vi "Craigslist Textbooks for Fusion Table V2.vi"() -> ()   [LabVIEW 2010]
uses:
  <vilib>/Utility/file.llb/Read From Spreadsheet File (string).vi
  <vilib>/Utility/file.llb/Write To Spreadsheet File (string).vi
panel:
  out "File Save Path":string
  out "Array":string[][](array[string])
  out "user books per city":string[][](array[string])
  out "Final filtered":string[][](array[string])
  out "element":string
  out "All closest city data":string[](array[string])
  out "All Data":string[][](array[string])
  out "ID number":string
  in  "Geo Locations 2":string[][](array[string])=[["http://boulder.craigslist.org/bks/", "http://boulder.craigslist.org/bks/index100.html", "http://boulder.craigslist.org/bks/index200.html", "http://boulder.craigslist.org/bks/index300.html", "http://boulder.craigslist.org/bks/index400.html", "http://boulder.craigslist.org/bks/index500.html", "http://boulder.craigslist.org/bks/index600.html", "http://boulder.craigslist.org/bks/index700.html", "http://boulder.craigslist.org/bks/index800.html", "http://boulder.craigslist.org/bks/index900.html", "40.006846", "-105.271575", "CU Boulder", "Boulder", "CO", "4/30/2004 7:48:47 PM", "3558694"], ["http://phoenix.craigslist.org/bks/", "http://phoenix.craigslist.org/bks/index100.html", "http://phoenix.craigslist.org/bks/index200.html", "http://phoenix.craigslist.org/bks/index300.html", "http://phoenix.craigslist.org/bks/index400.html", "http://phoenix.craigslist.org/bks/index500.html", "http://phoenix.craigslist.org/bks/index600.html", "http://phoenix.craigslist.org/bks/index700.html", "http://phoenix.craigslist.org/bks/index800.html", "http://phoenix.craigslist.org/bks/index900.html", "33.416147", "-111.938152", "ASU Arizona State University", "Phoenix", "AZ", "4/30/2004 7:48:47 PM", "3558688"], ["http://orlando.craigslist.org/bks/", "http://orlando.craigslist.org/bks/index100.html", "http://orlando.craigslist.org/bks/index200.html", "http://orlando.craigslist.org/bks/index300.html", "http://orlando.craigslist.org/bks/index400.html", "http://orlando.craigslist.org/bks/index500.html", "http://orlando.craigslist.org/bks/index600.html", "http://orlando.craigslist.org/bks/index700.html", "http://orlando.craigslist.org/bks/index800.html", "http://orlando.craigslist.org/bks/index900.html", "28.602326", "-81.19994", "UCF University of Central Florida", "orlando", "FL", "", "3558796"], ["http://austin.craigslist.org/bks/", "http://austin.craigslist.org/bks/index100.html", "http://austin.craigslist.org/bks/index200.html", "http://austin.craigslist.org/bks/index300.html", "http://austin.craigslist.org/bks/index400.html", "http://austin.craigslist.org/bks/index500.html", "http://austin.craigslist.org/bks/index600.html", "http://austin.craigslist.org/bks/index700.html", "http://austin.craigslist.org/bks/index800.html", "http://austin.craigslist.org/bks/index900.html", "30.28629", "-97.740211", "UT Austin University of Texas at Austin", "Austin", "TX", "40.006846", "3588692"], ["http://columbus.craigslist.org/bks/", "http://columbus.craigslist.org/bks/index100.html", "http://columbus.craigslist.org/bks/index200.html", "http:/columbus.craigslist.org/bks/index300.html", "http://columbus.craigslist.org/bks/index400.html", "http://columbus.craigslist.org/bks/index500.html", "http://columbus.craigslist.org/bks/index600.html", "http://columbus.craigslist.org/bks/index700.html", "http://columbus.craigslist.org/bks/index800.html", "http://columbus.craigslist.org/bks/index900.html", "40.000778", "-83.010421", "OSU Ohio State University", "Columbus", "OH", "4/30/2004 7:48:47 PM", "3558876"], ["http://minneapolis.craigslist.org/bks/", "http://minneapolis.craigslist.org/bks/index100.html", "http://minneapolis.craigslist.org/bks/index200.html", "http://minneapolis.craigslist.org/bks/index300.html", "http://minneapolis.craigslist.org/bks/index400.html", "http://minneapolis.craigslist.org/bks/index500.html", "http://minneapolis.craigslist.org/bks/index600.html", "http://minneapolis.craigslist.org/bks/index700.html", "http://minneapolis.craigslist.org/bks/index800.html", "http://minneapolis.craigslist.org/bks/index900.html", "44.974999", "-93.231847", "U of M University of Minnesota", "minneapolis", "MN", "", "3558694"], ["http://losangeles.craigslist.org/lac/bks/", "http://losangeles.craigslist.org/lac/bks/index100.html", "http://losangeles.craigslist.org/lac/bks/index200.html", "http://losangeles.craigslist.org/lac/bks/index300.html", "http://losangeles.craigslist.org/lac/bks/index400.html", "http://losangeles.craigslist.org/lac/bks/index500.html", "http://losangeles.craigslist.org/lac/bks/index600.html", "http://losangeles.craigslist.org/lac/bks/index700.html", "http://losangeles.craigslist.org/lac/bks/index800.html", "http://losangeles.craigslist.org/lac/bks/index900.html", "34.020612", "-118.284409", "USC University of Southern California", "USC", "CA", "40.006846", "3588399"], ["http://boston.craigslist.org/gbs/bks/", "http://boston.craigslist.org/gbs/bks/index100.html", "http://boston.craigslist.org/gbs/bks/index200.html", "http://boston.craigslist.org/gbs/bks/index300.html", "http://boston.craigslist.org/gbs/bks/index400.html", "http://boston.craigslist.org/gbs/bks/index500.html", "http://boston.craigslist.org/gbs/bks/index600.html", "http://boston.craigslist.org/gbs/bks/index700.html", "http://boston.craigslist.org/gbs/bks/index800.html", "http://boston.craigslist.org/gbs/bks/index900.html", "42.372852", "-71.117581", "Harvard University", "Cambridge", "MA", "40.006846", "3589108"], ["http://newhaven.craigslist.org/bks/", "http://newhaven.craigslist.org/bks/index100.html", "http://newhaven.craigslist.org/bks/index200.html", "http://newhaven.craigslist.org/bks/index300.html", "http://newhaven.craigslist.org/bks/index400.html", "http://newhaven.craigslist.org/bks/index500.html", "http://newhaven.craigslist.org/bks/index600.html", "http://newhaven.craigslist.org/bks/index700.html", "http://newhaven.craigslist.org/bks/index800.html", "http://newhaven.craigslist.org/bks/index900.html", "41.311211", "-72.928662", "Yale University", "New Haven", "CT", "40.006846", "3588844"], ["http://sfbay.craigslist.org/pen/bks/", "http://sfbay.craigslist.org/pen/bks/index100.html", "http://sfbay.craigslist.org/pen/bks/index200.html", "http://sfbay.craigslist.org/pen/bks/index300.html", "http://sfbay.craigslist.org/pen/bks/index400.html", "http://sfbay.craigslist.org/pen/bks/index500.html", "http://sfbay.craigslist.org/pen/bks/index600.html", "http://sfbay.craigslist.org/pen/bks/index700.html", "http://sfbay.craigslist.org/pen/index800.html", "http://sfbay.craigslist.org/pen/bks/index900.html", "37.425576", "-122.168891", "Stanford University", "Redwood City", "CA", "40.006846", "3588839"], ["http://chicago.craigslist.org/nch/bks/", "http://chicago.craigslist.org/nch/bks/index100.html", "http://chicago.craigslist.org/nch/bks/index200.html", "http://chicago.craigslist.org/nch/bks/index300.html", "http://chicago.craigslist.org/nch/bks/index400.html", "http://chicago.craigslist.org/nch/bks/index500.html", "http://chicago.craigslist.org/nch/bks/index600.html", "http://chicago.craigslist.org/nch/bks/index700.html", "http://chicago.craigslist.org/nch/bks/index800.html", "http://chicago.craigslist.org/nch/bks/index900.html", "42.057801", "-87.67563", "NU Northwestern University", "Evanston", "IL", "40.006846", "3588099"], ["http://sfbay.craigslist.org/eby/bks/", "http://sfbay.craigslist.org/eby/bks/index100.html", "http://sfbay.craigslist.org/eby/bks/index200.html", "http://sfbay.craigslist.org/eby/bks/index300.html", "http://sfbay.craigslist.org/eby/bks/index400.html", "http://sfbay.craigslist.org/eby/bks/index500.html", "http://sfbay.craigslist.org/eby/bks/index600.html", "http://sfbay.craigslist.org/eby/bks/index700.html", "http://sfbay.craigslist.org/eby/bks/index800.html", "http://sfbay.craigslist.org/eby/bks/index900.html", "37.872296", "-122.258799", "UC Berkeley University of California at Berkeley", "Berkeley", "CA", "40.006846", "3588671"], ["http://fortcollins.craigslist.org/bks/", "http://fortcollins.craigslist.org/bks/index100.html", "http://fortcollins.craigslist.org/bks/index200.html", "http://fortcollins.craigslist.org/bks/index300.html", "http://fortcollins.craigslist.org/bks/index400.html", "http://fortcollins.craigslist.org/bks/index500.html", "http://fortcollins.craigslist.org/bks/index600.html", "http://fortcollins.craigslist.org/bks/index700.html", "http://fortcollins.craigslist.org/bks/index800.html", "http://fortcollins.craigslist.org/bks/index900.html", "40.571556", "-105.080624", "CSU Colorado State University", "Fort Collins", "CO", "40.006846", "3589102"], ["http://denver.craigslist.org/bks/", "http://denver.craigslist.org/bks/index100.html", "http://denver.craigslist.org/bks/index200.html", "http://denver.craigslist.org/bks/index300.html", "http://denver.craigslist.org/bks/index400.html", "http://denver.craigslist.org/bks/index500.html", "http://denver.craigslist.org/bks/index600.html", "http://denver.craigslist.org/bks/index700.html", "http://denver.craigslist.org/bks/index800.html", "http://denver.craigslist.org/bks/index900.html", "39.676707", "-104.962628", "DU University of Denver", "Denver", "CO", "40.006846", "3588279"], ["http://boston.craigslist.org/gbs/bks/", "http://boston.craigslist.org/gbs/bks/index100.html", "http://boston.craigslist.org/gbs/bks/index200.html", "http://boston.craigslist.org/gbs/bks/index300.html", "http://boston.craigslist.org/gbs/bks/index400.html", "http://boston.craigslist.org/gbs/bks/index500.html", "http://boston.craigslist.org/gbs/bks/index600.html", "http://boston.craigslist.org/gbs/bks/index700.html", "http://boston.craigslist.org/gbs/bks/index800.html", "http://boston.craigslist.org/gbs/bks/index900.html", "42.361556", "-71.090759", "MIT Massachusetts Institute of Technology", "Cambridge", "MA", "40.006846", "3588278"]]
  out "Finished Array":string[][](array[string])
  out "One Row Edited":string[](array[string])
  out "Craigslist Link":string
  out "Place":string
  out "One Row Unedited":string[](array[string])
  out "Category":string
  out "Extra Information":string
  out "Price":string
  out "General Location":string
  out "Time":string
  out "Date":string
  out "Year":string
  out "Date, Time":string
  out "State":string
  out "City":string
  out "long string":string
  out "lat string":string
  out "Full Source":string
  out "long":dbl
  out "lat":dbl
  out "Body":string
  out "E-mail Contact":string
  out "Title":string
  out "Parse Count":i32
  out "Current Page Source":string
  # "http://thestudentbookproject.org/index2.php?option=com_google_maps_boulder&task=dynamic&no_html=1&download=true&zip=false"
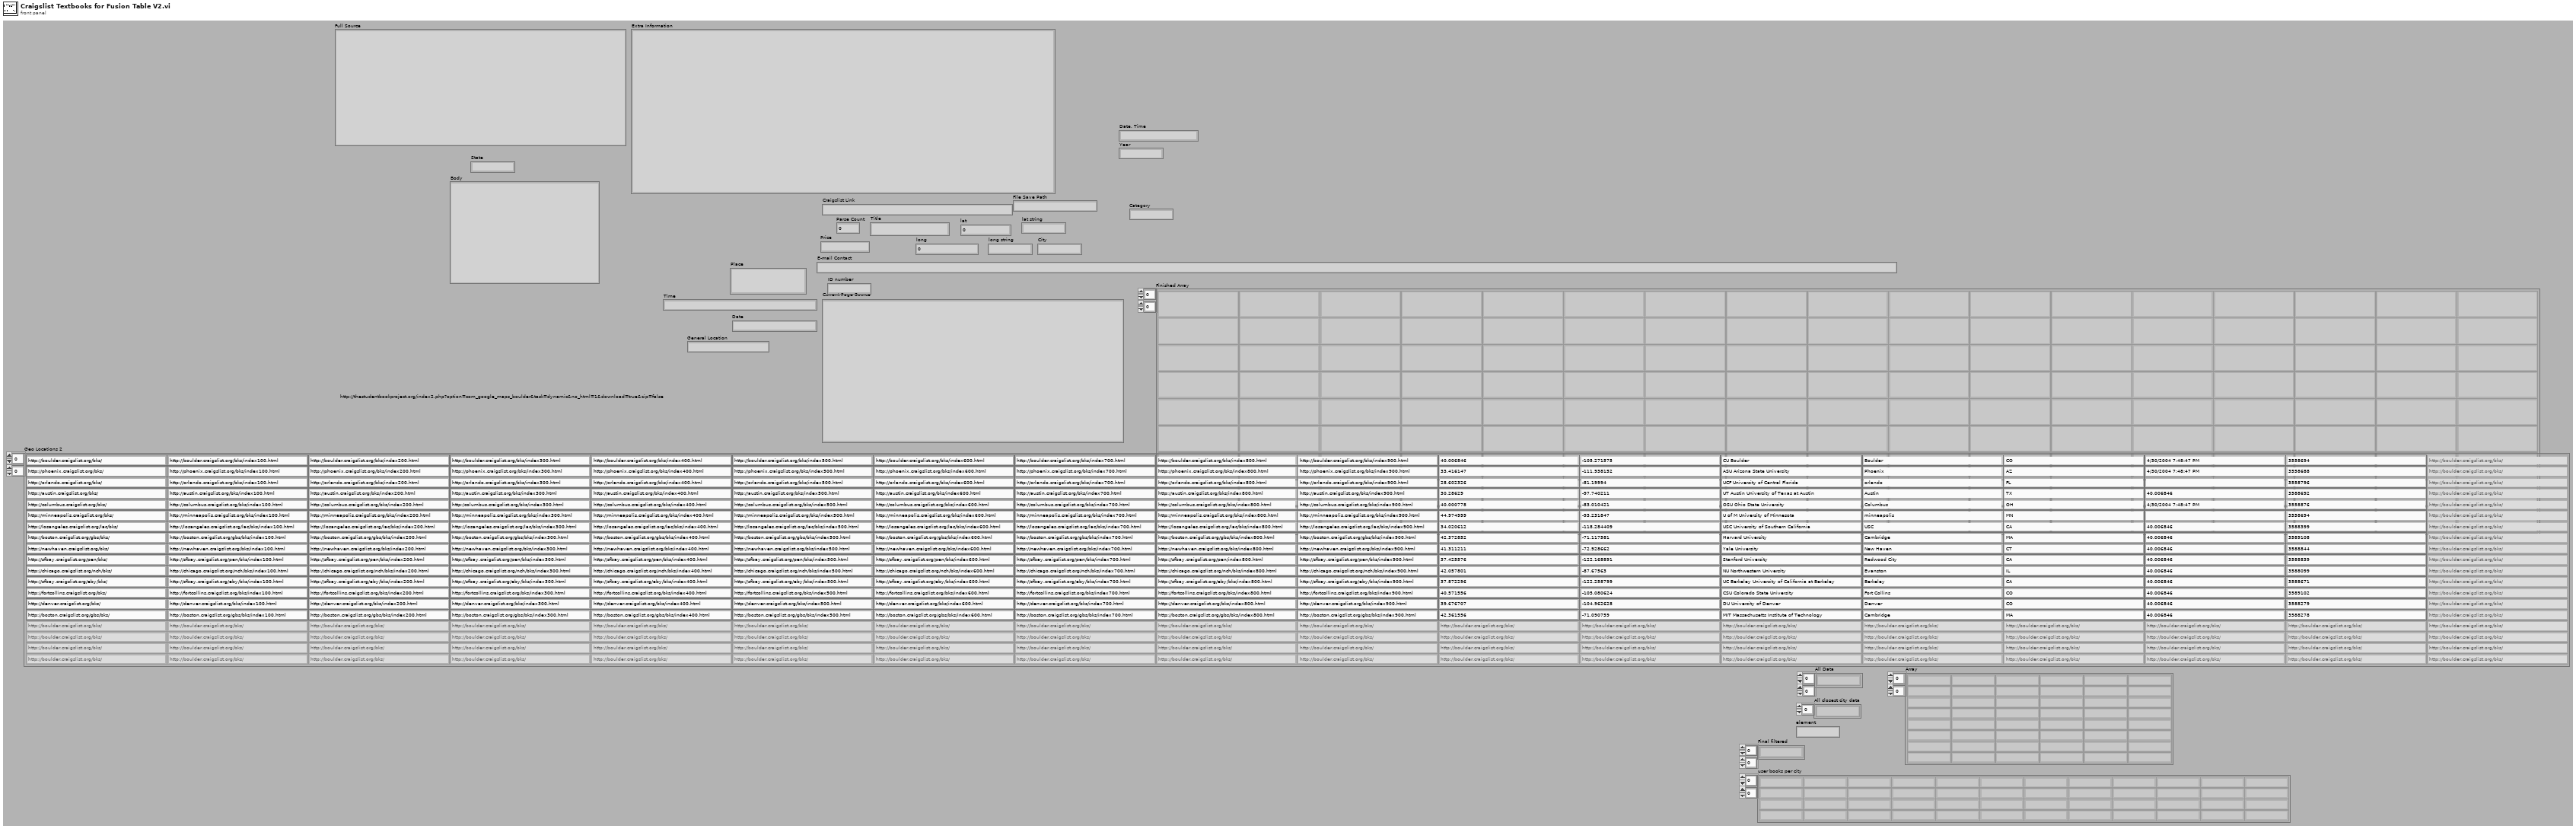
[diagram p1: front panel]
types:
  T1 = enum16{"open", "replace", "create", "open or create", "replace or create", "replace or create with confirmation"}
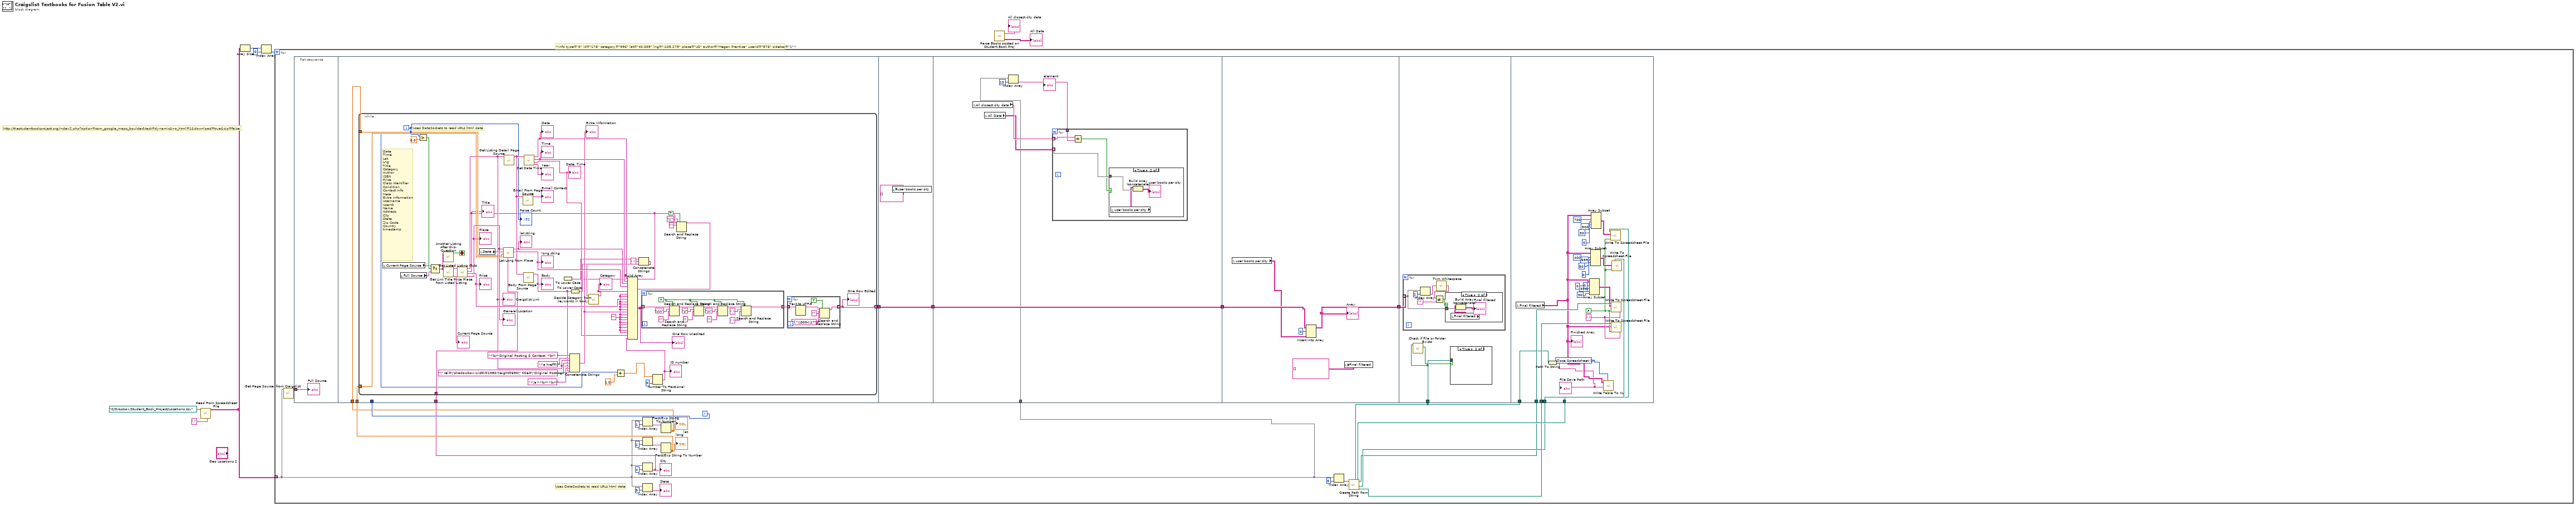
[diagram p0: block diagram]
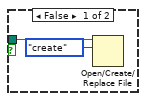
[diagram p3: hidden frame]
diagram:
  # "http://thestudentbookproject.org/index2.php?option=com_google_maps_boulder&task=dynamic&no_html=1&download=true&zip=false"
  # "<info type=\"0\" id=\"176\" category=\"996\" lat=\"40.005\" lng=\"-105.275\" place=\"US\" author=\"Megan Prentice\" userid=\"876\" sidebar=\"1\">"
  n1 = call-poly <vilib>:"Read From Spreadsheet File.vi"("delimiter (\\t)"="," ("delimiter (\\t)"), "file path (dialog if empty)"=path "C:/Dropbox/Student_Book_Project/Locations.csv") -> ("all rows"=w3:string[][])  [unwired: 5 in, 4 out]
  n2 = Array Size(array=w3) -> (size(s)=w8:i32[])
  n3 = Index Array(array=w8, index=0) -> (element=w6:i32)
  n4 = for {
    N: w6 -> [_]
    tunnel: w3 -> [w12] mode=indexing
    i -> [w24]
    # "Uses DataSockets to read URLs html data"
    n5 = call "Get Page Source  from Craigslist.vi"("Input Vaiables Array"=w12) -> ("Full Page Source of 9 pages combined"=w22:string)  [unwired: 10 in]
    n6 = flat-sequence {
      tunnel: w22 -> [w33]
      tunnel: w24 -> [_]
      tunnel: [w37] -> w11
      tunnel: w21 -> [w36]
      tunnel: w20 -> [w35]
      tunnel: w19 -> [w34]
      tunnel: w11 -> [w107]
      tunnel: [w107] -> w10
      tunnel: [w113] -> w13
      tunnel: w12 -> [w108]
      tunnel: w10 -> [w113]
      tunnel: w13 -> [w124]
      tunnel: [w121] -> w14
      tunnel: w14 -> [w128]
      tunnel: w9 -> [w127]
      tunnel: w9 -> [w143]
      tunnel: w16 -> [w147]
      tunnel: w17 -> [w148]
      tunnel: w15 -> [w162]
      tunnel: w23 -> [w163]
      frame #0 {
        "Full Source" <- w33
      }
      frame #1 {
        n7 = while {
          tunnel: [w57] -> w37 mode=indexing
          tunnel: w36 -> [w61]
          tunnel: w35 -> [w60]
          tunnel: w34 -> [w49]
          i -> [w46]
          stop <- w76 stop-if-true
          w77 = "" ("element")
          # "Date\nTime\nLat\nLng\nTitle\nCategory\nAuthor\nISBN\nPrice\nClass Identifier\nCondition\nContact Info\nMeta\nExtra Information\nUsername\nUserID\nName\nAddress\nCity\nState\nZip Code \nCountry\ntimestamp"
          # "Uses DataSockets to read URLs html data"
          n8 = local read "Current Page Source"() -> (w83:string)
          n9 = local read "Full Source"() -> (w82:string)
          n10 = Greater?(x=w46, y=0.0) -> (0:w84:bool)
          n11 = Select(t=w83, s=w84, f=w82) -> (s? t:f=w75:string)
          n12 = call "Another Listing After this- Question.vi"("Current Page Source"=w75) -> ("Another Listing After"=w76:bool)  [unwired: 10 in]
          n13 = call "Get Listed Listing Guts.vi"("Current Page Source"=w75) -> ("Updated Page Source"=→"Current Page Source":string, "Listed Listing Guts"=w73:string)  [unwired: 9 in]
          n14 = call "Get Link Title Price Place from Listed Listing.vi"("Listed Listing Guts"=w73) -> ("Place"=w71:string, "Price w/ $ sign"=w72:string, "Listing Title"=w42:string, "Craigslist Link"=w67:string)  [unwired: 7 in]
          "Title" <- w42
          "General Location" <- w71
          "Price" <- w72
          "Place" <- w71
          "Craigslist Link" <- w67
          n15 = local read "State"() -> (w70:string)
          n16 = call "Lat Long from Place.vi"("City default name"=w49, "Long"=w60, "Lat"=w61, "County/State"=w70, "CL Place Name"=w71) -> ("long string"=w68:string, "lat string"=w69:string)  [unwired: 5 in]
          "lat string" <- w69
          "long string" <- w68
          n17 = call "Get Listing Detail Page Source.vi"("URL"=w67) -> ("Page Source"=w65:string)  [unwired: 10 in]
          n18 = call "Email From Page Source.vi"("Detail Page Source"=w65) -> ("E-mail Contact"=→"E-mail Contact":string)  [unwired: 10 in]
          n19 = call "Body From Page Source.vi"("Detail Page Source"=w65) -> ("Body (Body, Images, Location, Everything)"=w63:string)  [unwired: 10 in]
          "Body" <- w63
          n20 = call "Get Date Time.vi"("Detail Page Source"=w65) -> ("Year"=→"Year":string, "Date, Time"=w54:string, "Time"=w55:string, "Date"=w56:string)  [unwired: 7 in]
          "Date, Time" <- w54
          "Date" <- w56
          "Time" <- w55
          n21 = To Lower Case(string=w42) -> (all lower case string=w53:string)
          n22 = Concatenate Strings("<br>Original Posting & Contact: <br> " ("string"), "<a href=\"" ("string"), w67, "\" rel=\"shadowbox;width=1380;height=690\" title=\"Original Posting\">" ("string"), w67, "</a><br><br>" ("string"), w63) -> (w62:string)
          "Extra Information" <- w62
          n23 = To Lower Case(string=w63) -> (all lower case string=w52:string)
          n24 = Add(x=w46, y=1.0) -> (x+y=w45:dbl)
          n25 = Concatenate Strings(w53, " " ("string"), w52) -> (w51:string)
          n26 = call "Decide Category from keywords in body.vi"("Body of Posting to Search"=w51) -> ("Category Determined"=w44:string)  [unwired: 10 in]
          "Category" <- w44
          n27 = Number To Fractional String(number=w45, precision (6)=i16 0) -> (F-format string=w47:string)  [unwired: 2 in]
          "ID number" <- w47
          n28 = Search and Replace String(replace all?=TRUE ("replace all? (F)"), input string=w42, search string="'", replace string="\\'" ("replace string (\"\")")) -> (result string=w39:string)  [unwired: 4 in, 3 out]
          n29 = Build Array(w56, w55, w69, w68, w39, w44, w77, w77, w72, w77, w77, w77, w77, w62, w77, w77, w77, w77, w77, w77, w77, w77, w54, w47) -> (w59:string[])
          "One Row Unedited" <- w59
          n30 = for {
            tunnel: w59 -> [w105] mode=indexing
            tunnel: [w92] -> w58 mode=indexing
            w93 = TRUE ("replace all? (F)")
            n31 = Search and Replace String(replace all?=w93, input string=w105, search string="\r\n", replace string="" ("replace string (\"\")")) -> (result string=w100:string)  [unwired: 4 in, 3 out]
            n32 = Search and Replace String(replace all?=w93, input string=w100, search string="\r", replace string="" ("replace string (\"\")")) -> (result string=w99:string)  [unwired: 4 in, 3 out]
            n33 = Search and Replace String(replace all?=w93, input string=w99, search string="\n", replace string="" ("replace string (\"\")")) -> (result string=w94:string)  [unwired: 4 in, 3 out]
            n34 = Search and Replace String(replace all?=w93, input string=w94, search string=",", replace string=" " ("replace string (\"\")")) -> (result string=w92:string)  [unwired: 4 in, 3 out]
          }
          n35 = for {
            tunnel: w58 -> [w91] mode=indexing
            tunnel: [w88] -> w57 mode=indexing
            n36 = Text to UTF-8(11:w91) -> (3:w89:string)  [unwired: 1 in, 1 out]
            n37 = Search and Replace String(replace all?=TRUE ("replace all? (F)"), input string=w89, search string="[^\\000-\\177]", replace string="" ("replace string (\"\")")) -> (result string=w88:string)  [unwired: 4 in, 3 out]
          }
          "One Row Edited" <- w57
          "Parse Count" <- w46
        }
      }
      frame #2 {
        n38 = local write "user books per city"(string[][] [] ("user books per city")) -> ()
      }
      frame #3 {
        n39 = local read "All closest city data"() -> (w111:string[])
        n40 = local read "All Data"() -> (w109:string[][])
        n41 = Index Array(array=w108, index=13) -> (element=w110:string)
        "element" <- w110
        n42 = for {
          tunnel: w111 -> [w117] mode=indexing
          tunnel: w110 -> [w116]
          tunnel: w109 -> [w115] mode=indexing
          n43 = Equal?(x=w117, y=w116) -> (x = y?=w114:bool)
          n44 = case shown="True" w114 {
            tunnel: w115 -> [_ w120]
            frame False {
            }
            frame True {
              n45 = local read "user books per city"() -> (w118:string[][])
              n46 = Build Array (concatenate)(w118, w120) -> (→"user books per city":string[][])
            }
          }
        }
      }
      frame #4 {
        n47 = local read "user books per city"() -> (w122:string[][])
        n48 = Insert Into Array(array=w124, index (row)=0, new element=w122) -> (w121:string[][])  [unwired: 1 in]
        "Array" <- w121
        n49 = local write "Final filtered"(string[][] [] ("Final filtered")) -> ()
      }
      frame #5 {
        n50 = for {
          tunnel: w128 -> [w134] mode=indexing
          n51 = Index Array(array=w134, index=2) -> (element=w133:string)
          n52 = call <vilib>:"Trim Whitespace.vi"("string"=w133) -> ("trimmed string"=w132:string)  [unwired: 1 in]
          n53 = Not Equal?(x=w132, y="") -> (x != y?=w135:bool)
          n54 = case shown="True" w135 {
            tunnel: w134 -> [_ w139]
            frame False {
            }
            frame True {
              n55 = local read "Final filtered"() -> (w137:string[][])
              n56 = Build Array (concatenate)(w137, w139) -> (→"Final filtered":string[][])
            }
          }
        }
        n57 = call <vilib>:"Check if File or Folder Exists.vi"("path"=w127) -> ("file or folder exists?"=w126:bool)  [unwired: 8 in, 2 out]
        n58 = case shown="True" w126 {
          tunnel: w127 -> [w129 _]
          frame False {
            n59 = Open/Create/Replace File(file path (use dialog)=w129, operation (0:open)=T1."create") -> ()  [unwired: 4 in, 3 out]
          }
          frame True {
          }
        }
      }
      frame #6 {
        w142 = u16 1 items=["Leave Excel Open", "Close Spreadsheet"] ("Completion Task")
        w145 = FALSE ("append to file? (new file:F)")
        w144 = "," ("delimiter (\\t)")
        n60 = local read "Final filtered"() -> (w141:string[][])
        "Finished Array" <- w141
        n61 = Path To String(path=w143) -> (string=w140:string)
        "File Save Path" <- w140
        n62 = Array Subset(array=w141, index (row)=0 ("index"), length (row)=399 ("length"), index (col)=0 ("index"), length (col)=30 ("length")) -> (w157:string[][])
        n63 = Array Subset(array=w141, index (row)=400 ("index"), length (row)=699 ("length"), index (col)=0 ("index"), length (col)=30 ("length")) -> (w164:string[][])
        n64 = Array Subset(array=w141, index (row)=700 ("index"), length (row)=900 ("length"), index (col)=0 ("index"), length (col)=30 ("length")) -> (w146:string[][])
        n65 = call "Write Table To XL.vi"("Table"=w141, "Filename"=w140, "Completion Task"=w142) -> ()  [unwired: 4 in]
        n66 = call-poly <vilib>:"Write To Spreadsheet File.vi"("append to file? (new file:F)"=w145, "2D data"=w146, "file path (dialog if empty)"=w147) -> ()  [unwired: 5 in, 1 out]
        n67 = call-poly <vilib>:"Write To Spreadsheet File.vi"("delimiter (\\t)"=w144, "append to file? (new file:F)"=w145, "2D data"=w157, "file path (dialog if empty)"=w162) -> ()  [unwired: 4 in, 1 out]
        n68 = call-poly <vilib>:"Write To Spreadsheet File.vi"("delimiter (\\t)"=w144, "append to file? (new file:F)"=w145, "2D data"=w141, "file path (dialog if empty)"=w163) -> ()  [unwired: 4 in, 1 out]
        n69 = call-poly <vilib>:"Write To Spreadsheet File.vi"("append to file? (new file:F)"=w145, "2D data"=w164, "file path (dialog if empty)"=w148) -> ()  [unwired: 5 in, 1 out]
      }
    }
    n70 = Index Array(array=w12, index=1) -> (element=w30:string)
    n71 = Index Array(array=w12, index=2) -> (element=w29:string)
    n72 = Index Array(array=w12, index=4) -> (element=w19:string)
    "City" <- w19
    n73 = Index Array(array=w12, index=5) -> (element=→"State":string)
    n74 = Fract/Exp String To Number(string=w30) -> (number=w21:dbl)  [unwired: 3 in, 1 out]
    "lat" <- w21
    n75 = Fract/Exp String To Number(string=w29) -> (number=w20:dbl)  [unwired: 3 in, 1 out]
    "long" <- w20
    n76 = Index Array(array=w12, index=3) -> (element=w18:string)
    n77 = call "Create Path from String.vi"("Folder Name (CU Boulder)"=w18) -> ("Permanent Path"=w23:path, "Current Path 3"=w16:path, "Current Path 2"=w17:path, "Current Path"=w15:path, "Google Docs Path"=w9:path)  [unwired: 6 in]
  }
  n78 = call "Parse Books posted on Student Book Proj.vi"() -> ("All Data"=→"All Data":string[][], "All closest city data"=→"All closest city data":string[])  [unwired: 2 in]
